vi "NI CLI Add.vi"(11 "Inputs":string[](array[string])) -> (2 "Output/Failure":string, 3 "CLI Process Return Code":i32)   [LabVIEW 2014]
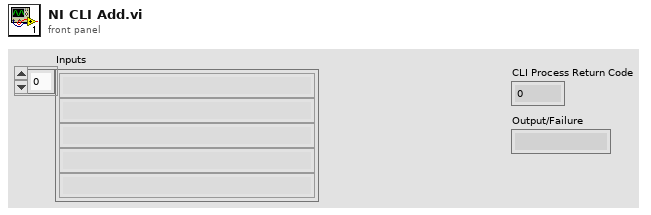
[diagram p1: front panel]
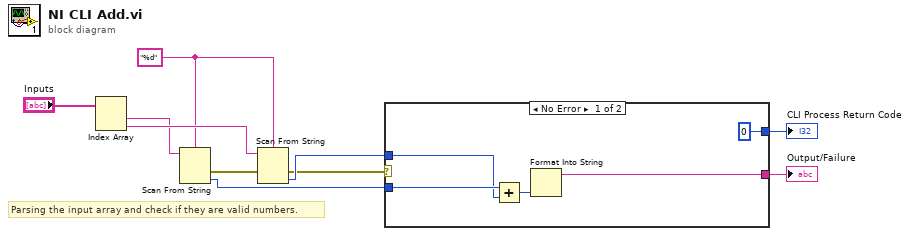
[diagram p0: block diagram]
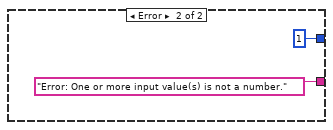
[diagram p2: hidden frame]
diagram:
  w8 = "%d" ("format string")
  # "Parsing the input array and check if they are valid numbers."
  n1 = Index Array "Index Array"(array="Inputs") -> (element #1=w3:string, element #2=w9:string)  [unwired: 2 in]
  n2 = Scan From String(format string=w8, input string=w3) -> (error out=w5:errorcluster, output 1=w6:i32)  [unwired: 3 in, 2 out]
  n3 = Scan From String(format string=w8, input string=w9, error in=w5) -> (error out=w4:errorcluster, output 1=w7:i32)  [unwired: 2 in, 2 out]
  n4 = case shown="No Error" w4 {
    tunnel: [0 1] -> w1
    tunnel: [w11 "Error: One or more input value(s) is not a number."] -> w2
    tunnel: w7 -> [w13 _]
    tunnel: w6 -> [w14 _]
    frame No Error {
      n5 = Add(x=w14, y=w13) -> (x+y=w12:i32)
      n6 = Format Into String(w12) -> (resulting string=w11:string)  [unwired: 3 in, 1 out]
    }
    frame Error {
    }
  }
  "CLI Process Return Code" <- w1
  "Output/Failure" <- w2
